vi "Set Brower Controls and VI Refnum.vi"(8 "error in (no error)":errorcluster, 10 "Brower Controls and VI Refnum":T1, 11 "Brower View in":refnum<class "Brower View.lvclass">) -> (0 "error out":errorcluster, 3 "Brower View out":refnum<class "Brower View.lvclass">)   [LabVIEW 2015, in "Brower View.lvclass"]
uses:
  Brower View.lvclass
  Type Definition/Brower Controls and VI Refnum.ctl
  Brower View.lvclass/Brower View.ctl
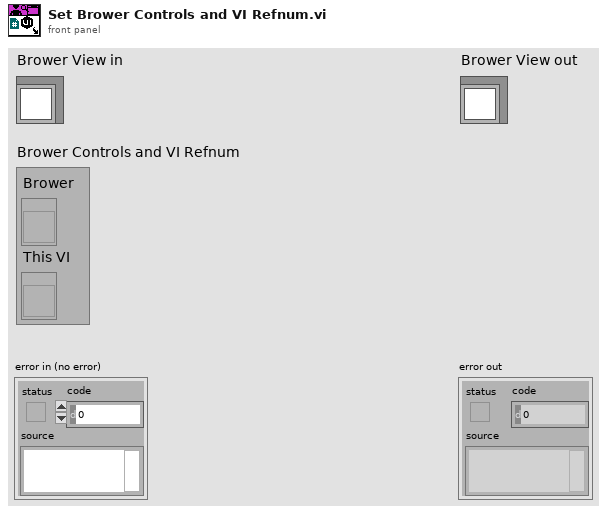
[diagram p1: front panel]
types:
  T1 = typedef "Brower View.lvclass/Brower Controls and VI Refnum.ctl" = cluster{"Brower":refnum<vi>, "This VI":refnum<vi>}
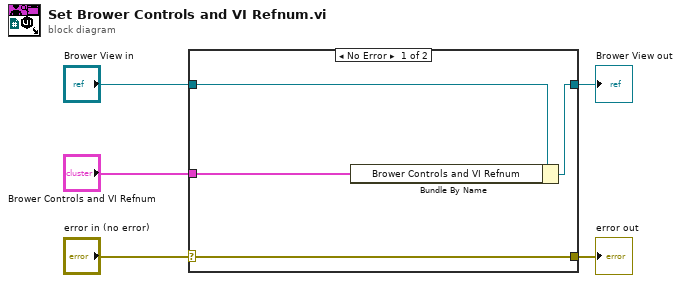
[diagram p0: block diagram]
diagram:
  n1 = case shown="No Error" "error in (no error)" {
    selector: "error in (no error)" -> [w9 w10]
    tunnel: [w9 w10] -> w4
    tunnel: [w7 w11] -> w2
    tunnel: "Brower View in" -> [w8 w11]
    tunnel: "Brower Controls and VI Refnum" -> [w6 _]
    frame No Error {
      n2 = Bundle By Name(cluster=w8, "Brower Controls and VI Refnum"=w6) -> (w7:refnum<class "Brower View.lvclass">)
    }
    frame Error {
    }
  }
  "error out" <- w4
  "Brower View out" <- w2
